vi "_Test Initialize Executor.vi"() -> ()   [LabVIEW 2021]
uses:
  Def-ExecutorConfigurations.ctl
  Typedef/Def-LogSpec.ctl
  Typedef/Def-CAN Port Configuration.ctl
  Typedef/Def-Executor Command.ctl
  XNET-CAN-Signal-Logger.lvlib
panel:
  out "value":T1={"LogSpec"={"Log file folder"=path "C:/Users/NI/Desktop/Data", "Log file name"="LogFile_{Year}-{Month}-{Day}-{Hour}-{Minute}-{Second}.tdms", "Segment Files"=FALSE, "Segment File Size"=100}, "CAN Configurations"=[]} {"LogSpec"."Segment File Size" format="%.0f MB"; "CAN Configurations"."Sample Rate (Hz)" format="%#_13g"}
  in  "stop":bool
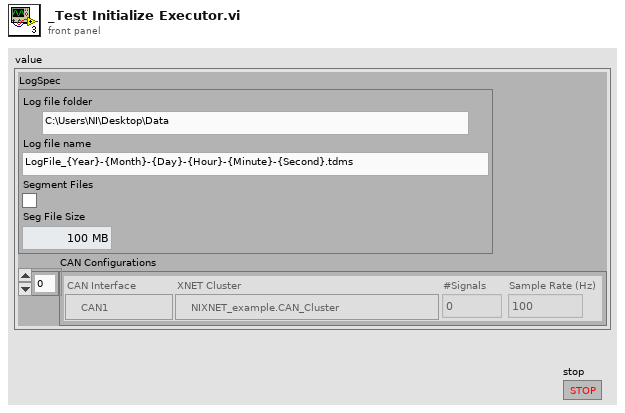
[diagram p1: front panel]
types:
  T1 = typedef "XNET-CAN-Signal-Logger.lvlib/Def-ExecutorConfigurations.ctl" = cluster{"LogSpec":T2, "CAN Configurations":T3[]}
  T2 = typedef "XNET-CAN-Signal-Logger.lvlib/Def-LogSpec.ctl" = cluster{"Log file folder":path, "Log file name":string, "Segment Files":bool, "Segment File Size":i64}
  T3 = typedef "XNET-CAN-Signal-Logger.lvlib/Def-CAN Port Configuration.ctl" = cluster{"CAN Interface":refnum<k21>, "XNET Cluster":refnum<k21>, "#Signals":i32, "Sample Rate (Hz)":dbl}
  T4 = typedef "XNET-CAN-Signal-Logger.lvlib/Def-Executor Command.ctl" = cluster{"Command":string, "Data":variant}
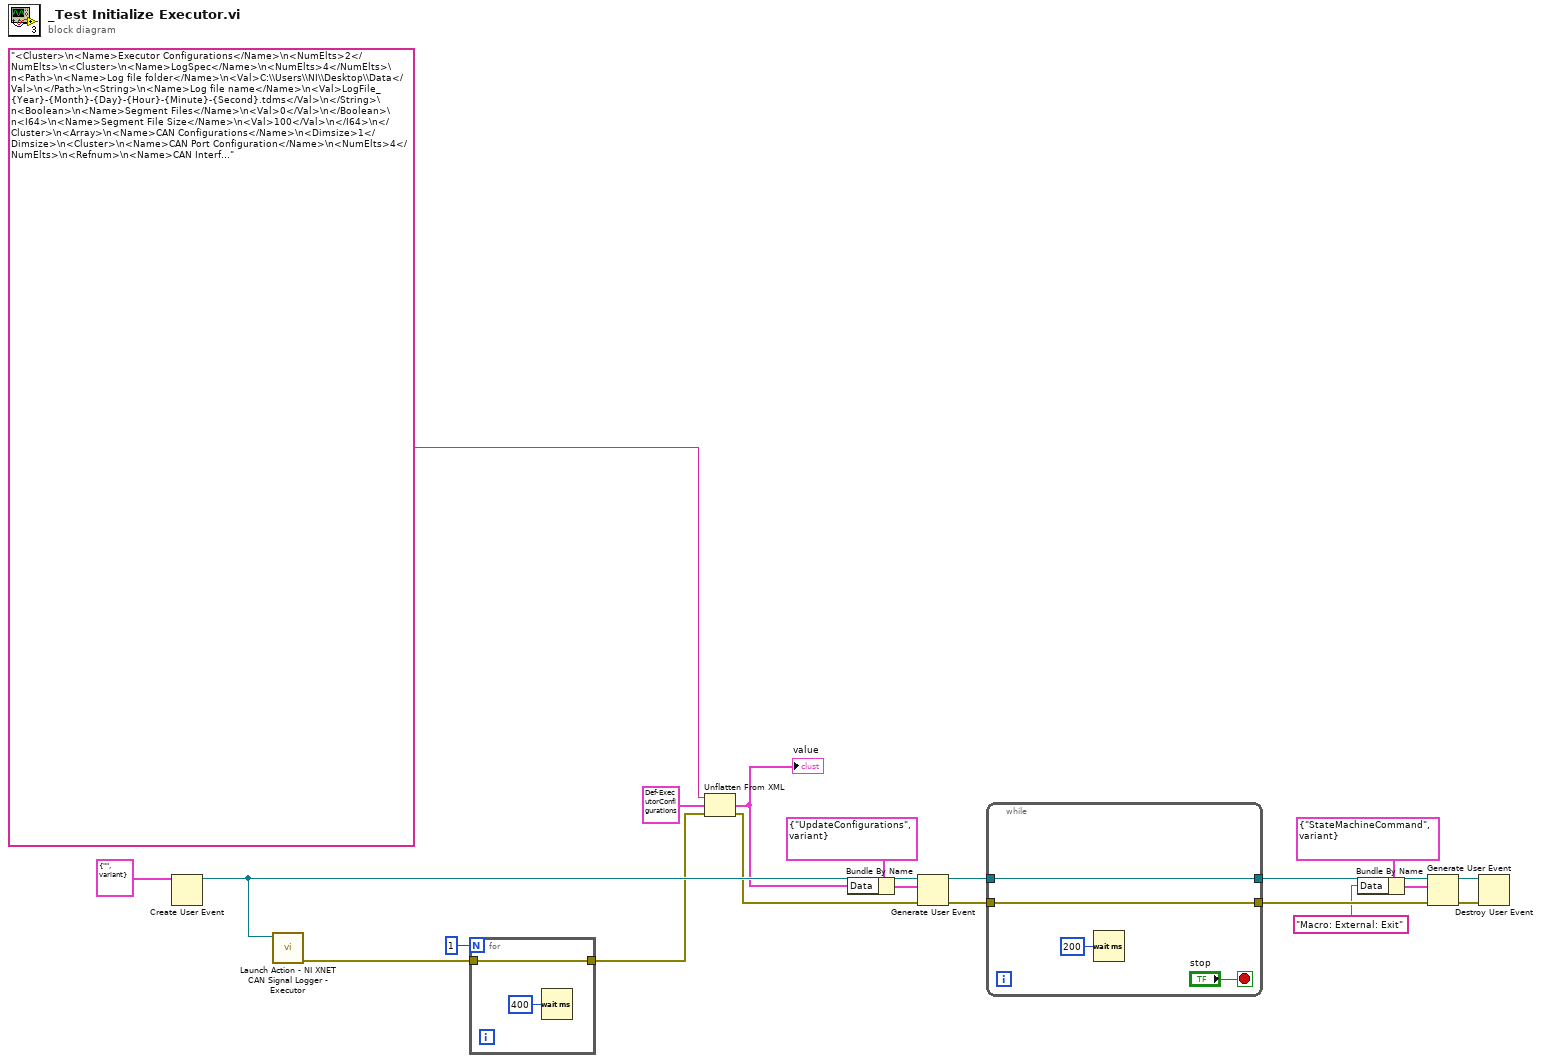
[diagram p0: block diagram]
diagram:
  n1 = Create User Event(user event datatype=T4 {"Command"="", "Data"=variant} ("Command")) -> (user event=w19:refnum<user-event>)  [unwired: 1 in, 1 out]
  n2 = call "Launch Action - NI XNET CAN Signal Logger - Executor.vi"("Executor Command"=w19) -> ("error out"=w10:errorcluster)  [unwired: 10 in]
  n3 = for {
    N: 1 -> [_]
    tunnel: [w21] -> w9
    tunnel: w10 -> [w21]
    n4 = Wait (ms)(milliseconds to wait=u32 400) -> ()  [unwired: 1 out]
  }
  n5 = Unflatten From XML(xml string="<Cluster>\n<Name>Executor Configurations</Name>\n<NumElts>2</NumElts>\n<Cluster>\n<Name>LogSpec</Name>\n<NumElts>4</NumElts>\n<Path>\n<Name>Log file folder</Name>\n<Val>C:\\Users\\NI\\Desktop\\Data</Val>\n</Path>\n<String>\n<Name>Log file name</Name>\n<Val>LogFile_{Year}-{Month}-{Day}-{Hour}-{Minute}-{Second}.tdms</Val>\n</String>\n<Boolean>\n<Name>Segment Files</Name>\n<Val>0</Val>\n</Boolean>\n<I64>\n<Name>Segment File Size</Name>\n<Val>100</Val>\n</I64>\n</Cluster>\n<Array>\n<Name>CAN Configurations</Name>\n<Dimsize>1</Dimsize>\n<Cluster>\n<Name>CAN Port Configuration</Name>\n<NumElts>4</NumElts>\n<Refnum>\n<Name>CAN Interface</Name>\n<RefKind>Generic Tag</RefKind>\n<RefType>xnet</RefType>\n<Val>CAN1</Val>\n</Refnum>\n<Refnum>\n<Name>XNET Cluster</Name>\n<RefKind>Generic Tag</RefKind>\n<RefType>xnet</RefType>\n<Val>NIXNET_example.CAN_Cluster</Val>\n</Refnum>\n<I32>\n<Name>#Signals</Name>\n<Val>28</Val>\n</I32>\n<DBL>\n<Name>Sample Rate (Hz)</Name>\n<Val>100.00000000000000</Val>\n</DBL>\n</Cluster>\n</Array>\n</Cluster>\n" ("Name"), type=T1 {"LogSpec"={"Log file folder"=path "C:/Users/NI/Desktop/Data", "Log file name"="LogFile_{Year}-{Month}-{Day}-{Hour}-{Minute}-{Second}.tdms", "Segment Files"=FALSE, "Segment File Size"=100}, "CAN Configurations"=[]} ("Executor Configurations"), error in (no error)=w9) -> (value=w14:T1, error out=w15:errorcluster)
  "value" <- w14
  n6 = Bundle By Name(cluster=T4 {"Command"="UpdateConfigurations", "Data"=variant} ("event data"), "Data"=w14) -> (w17:T4)
  n7 = Generate User Event(user event=w19, event data cluster=w17, error in=w15) -> (user event out=w12:refnum<user-event>, error out=w11:errorcluster)  [unwired: 1 in]
  n8 = while {
    tunnel: [w25] -> w6
    tunnel: w12 -> [w25]
    tunnel: [w23] -> w4
    tunnel: w11 -> [w23]
    stop <- "stop" stop-if-true
    n9 = Wait (ms)(milliseconds to wait=u32 200) -> ()  [unwired: 1 out]
  }
  n10 = Bundle By Name(cluster=T4 {"Command"="StateMachineCommand", "Data"=variant} ("event data"), "Data"="Macro: External: Exit") -> (w8:T4)
  n11 = Generate User Event(user event=w6, event data cluster=w8, error in=w4) -> (user event out=w5:refnum<user-event>, error out=w3:errorcluster)  [unwired: 1 in]
  n12 = Destroy User Event(user event=w5, error in=w3) -> ()  [unwired: 1 out]
